vi "圆环有无定位转换.vi"(8 "error in (no error)":errorcluster caption="错误输入（无错误）", 9 "Fitted Circle (定位)":T3 {"Average SNR (dB)" format="%.2f"; "Average Strength" format="%.2f"; "Roundness (Real-World)" format="%.2f"; "Radius (Real-World)" format="%.2f"; "Center (Real-World)"."Y" format="%.2f"; "Center (Real-World)"."X" format="%.2f"; "Radius (Pixels)" format="%.2f"; "Center (Pixels)"."Y" format="%.2f"; "Center (Pixels)"."X" format="%.2f"}, 10 "圆环ROI设定 in":T2 {"End Angle" min=-90.0 max=90.0 step=1.0 format="%.2f"; "Start Angle" min=-90.0 max=90.0 step=1.0 format="%.2f"; "Center X" scale=0.0..1024.0}, 11 "Image in":T1(plugin-control)) -> (0 "error out":errorcluster caption="错误输出", 1 "有无定位":bool, 2 "圆环ROI设定 out":T2 {"End Angle" min=-90.0 max=90.0 step=1.0 format="%.2f"; "Start Angle" min=-90.0 max=90.0 step=1.0 format="%.2f"; "Center X" scale=0.0..1024.0}, 3 "Image out":T1(plugin-control))   [LabVIEW 2017]
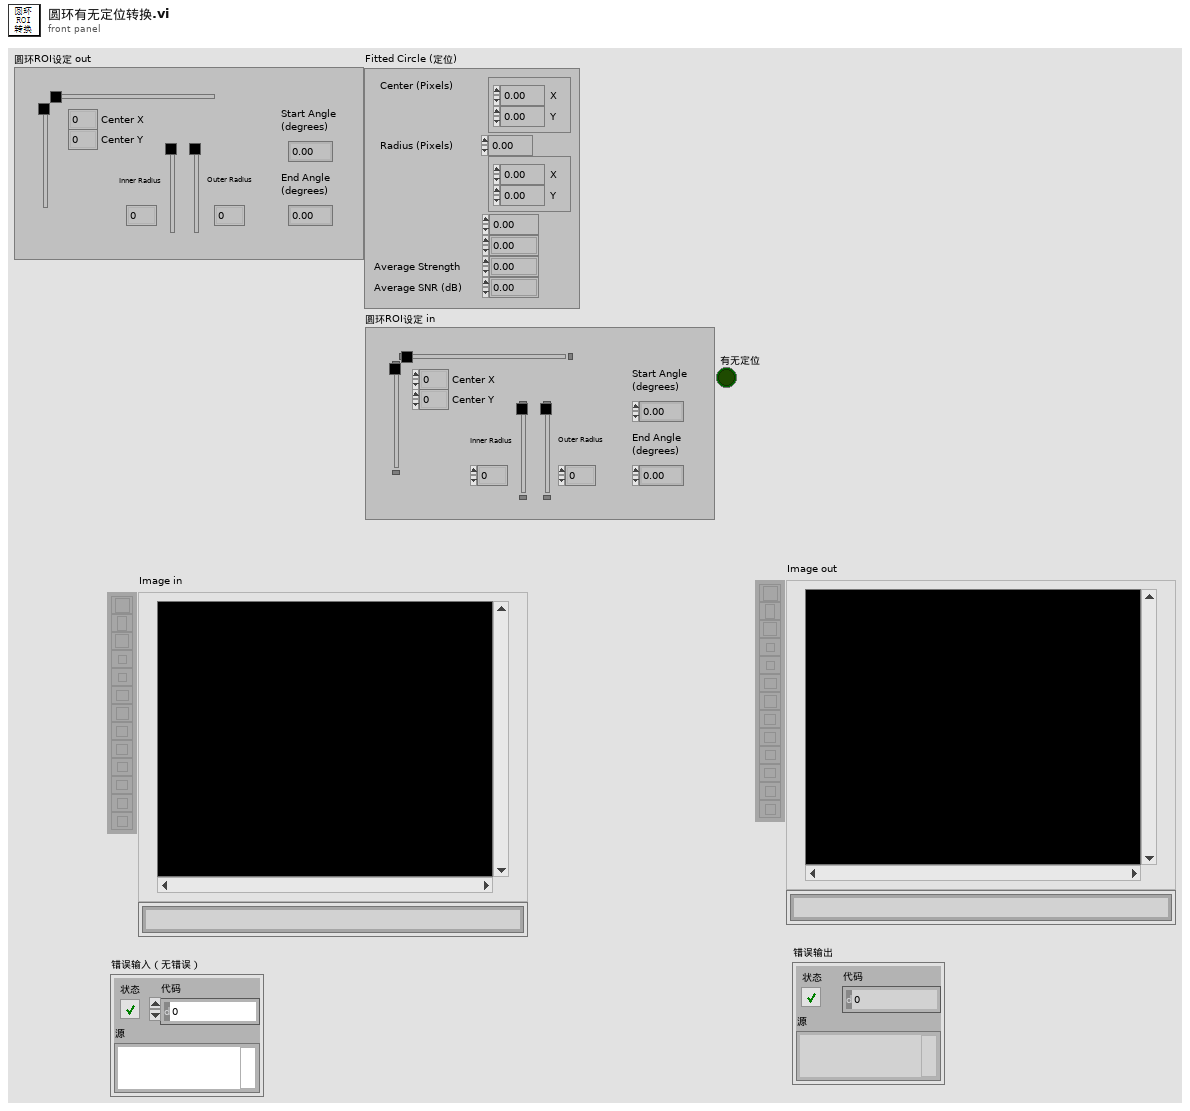
[diagram p1: front panel]
types:
  T1 = typedef "IMAQ Image.ctl" = refnum<image>
  T2 = typedef "IMAQ Circle" = cluster{"Center X":i32, "Center Y":i32, "Inner Radius":i32, "Outer Radius":i32, "Start Angle":dbl, "End Angle":dbl}
  T3 = cluster{"Center (Pixels)":cluster{"X":sgl, "Y":sgl}, "Radius (Pixels)":dbl, "Center (Real-World)":cluster{"X":sgl, "Y":sgl}, "Radius (Real-World)":dbl, "Roundness (Real-World)":dbl, "Average Strength":dbl, "Average SNR (dB)":dbl}
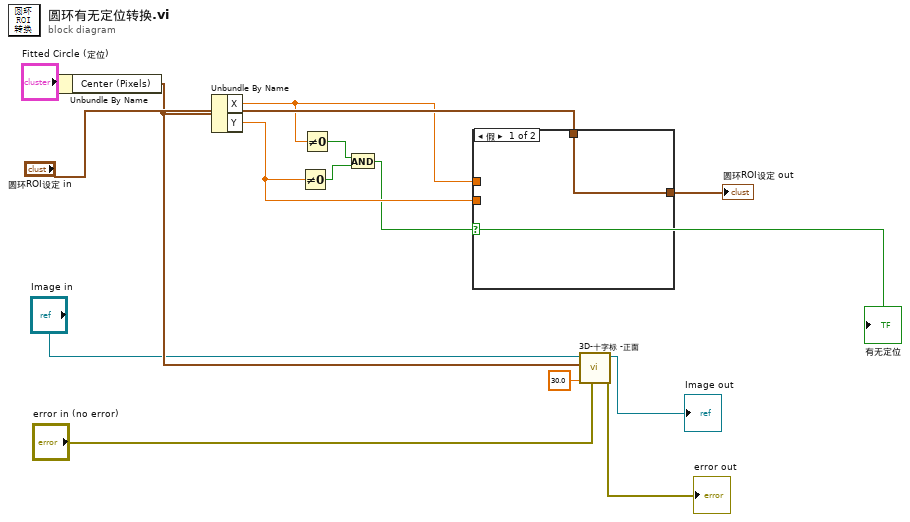
[diagram p0: block diagram]
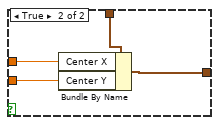
[diagram p2: hidden frame]
diagram:
  n1 = Unbundle By Name("Fitted Circle (定位)") -> ("Center (Pixels)"=w11:cluster{"X":sgl, "Y":sgl})
  n2 = Unbundle By Name(w11) -> ("X"=w5:sgl, "Y"=w4:sgl)
  n3 = Not Equal To 0?(x=w4) -> (x != 0?=w2:bool)
  n4 = Not Equal To 0?(x=w5) -> (x != 0?=w3:bool)
  n5 = And(x=w3, y=w2) -> (x .and. y?=w1:bool)
  "有无定位" <- w1
  n6 = case shown="假" w1 {
    tunnel: "圆环ROI设定 in" -> [w15 w19]
    tunnel: [w15 w18] -> w13
    tunnel: w5 -> [_ w17]
    tunnel: w4 -> [_ w16]
    frame False {
    }
    frame True {
      n7 = Bundle By Name(cluster=w19, "Center X"=w17, "Center Y"=w16) -> (w18:T2)
    }
  }
  "圆环ROI设定 out" <- w13
  n8 = call "3D-十字标 -正面.vi"("error in (no error)"="error in (no error)", "radius"=30.0, "Target Point"=w11, "输入图片"="Image in") -> ("error out"=→"error out":errorcluster, "输出图片"=→"Image out":T1)  [unwired: 6 in]
